vi "Agilent 33XXX Series Generate Frequency Sweep.vi"() -> ()   [LabVIEW 2010]
doc: "Shows how to configure and enable a frequency sweep."
uses:
  <instrlib>/Agilent 33XXX Series/Agilent 33XXX Series.lvlib
panel:
  in  "Serial Configuration":T1={"Baud Rate"=9600, "Parity"=0, "Data Bits"=8, "Flow Control"=4} {"Flow Control" items=["None", "XON/XOFF", "RTS/CTS", "XON/XOFF & RTS/CTS", "DTR/DSR", "XON/XOFF & DTR/DSR"]; "Data Bits" items=["7"=7, "8"=8]; "Parity" items=["None", "Odd", "Even", "Mark", "Space"]; "Baud Rate" items=["300"=300, "600"=600, "1200"=1200, "2400"=2400, "4800"=4800, "9600"=9600, "19200"=19200]}
  in  "Stop  Frequency (1000.0 Hz)":dbl=1000.0 format="%#.6g"
  in  "Start Frequency (100.0 Hz)":dbl=100.0 format="%#.6g"
  in  "Sweep Time (1.00 s)":dbl=1.0 format="%#.6g"
  in  "Amplitude (1 Vpp)":dbl=1.0
  in  "Waveform Function (1: Sine)":u16(ring)=1 items=["DC", "Sine", "Square", "Triangle", "Ramp", "Pulse", "Noise", "Sinc", "Negative Ramp", "Exponential Rise", "Exponential Fall", "Cardiac"]
  in  "VISA resource name":refnum<visa-resource-name>
  # "(c) 2008 National Instruments.  ALL RIGHTS RESERVED."
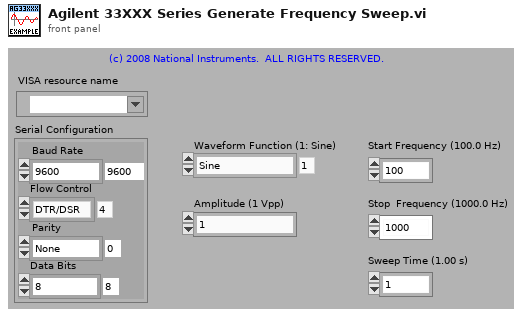
[diagram p1: front panel]
types:
  T1 = cluster{"Baud Rate":u32, "Parity":u16, "Data Bits":u16, "Flow Control":u16}
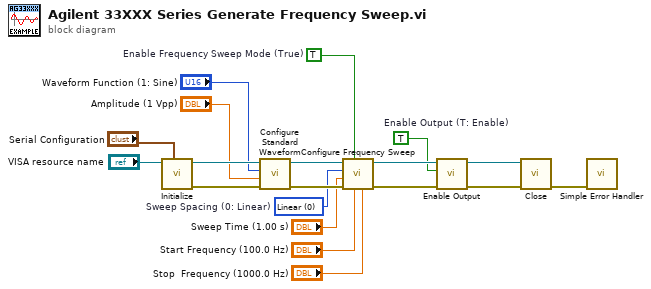
[diagram p0: block diagram]
diagram:
  w2 = u16 0 items=["Linear", "Logarithmic"]  # Sweep Spacing (0: Linear)
  w5 = TRUE  # Enable Output (T: Enable)
  w12 = TRUE  # Enable Frequency Sweep Mode (True)
  n1 = call <instrlib>:"Initialize.vi"("Serial Configuration"="Serial Configuration", "VISA resource name"="VISA resource name") -> ("error out"=w14:errorcluster, "VISA resource name out"=w19:refnum<visa-resource-name>)  [unwired: 8 in]
  n2 = call <instrlib>:"Configure Standard Waveform.vi"("error in (no error)"=w14, "Amplitude (1)"="Amplitude (1 Vpp)", "Waveform Function (1: Sine)"="Waveform Function (1: Sine)", "VISA resource name"=w19) -> ("error out"=w17:errorcluster, "VISA resource name out"=w16:refnum<visa-resource-name>)  [unwired: 6 in]
  n3 = call <instrlib>:"Configure Frequency Sweep.vi"("Stop  Frequency (1000.0 Hz)"="Stop  Frequency (1000.0 Hz)", "Start Frequency (100.0 Hz)"="Start Frequency (100.0 Hz)", "Enable Frequency Sweep Mode (T: Enable)"=w12, "error in (no error)"=w17, "Sweep Time (1.00 s)"="Sweep Time (1.00 s)", "Sweep Spacing (0: Linear)"=w2, "VISA resource name"=w16) -> ("error out"=w6:errorcluster, "VISA resource name out"=w7:refnum<visa-resource-name>)  [unwired: 3 in]
  n4 = call <instrlib>:"Enable Output.vi"("error in (no error)"=w6, "Enable Output  (T: Enable)"=w5, "VISA resource name"=w7) -> ("error out"=w3:errorcluster, "VISA resource name out"=w4:refnum<visa-resource-name>)  [unwired: 7 in]
  n5 = call <instrlib>:"Close.vi"("error in (no error)"=w3, "VISA resource name"=w4) -> ("error out"=w18:errorcluster)  [unwired: 9 in]
  n6 = call <vilib>:"Simple Error Handler.vi"("error in (no error)"=w18) -> ()  [unwired: 4 in, 5 out]
